vi "SimpleTokenizer.vi"() -> ()   [LabVIEW 2012]
uses:
  <vilib>/regexp/Match Regular Expression.xnode
panel:
  in  "Input String":string
  out "Next String Start":dbl
  out "Tokenized Array":string[](array[string])
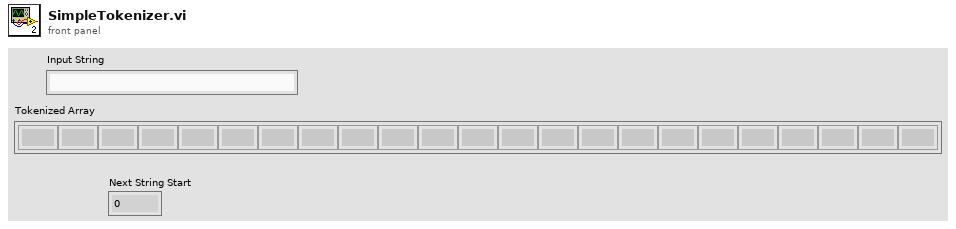
[diagram p1: front panel]
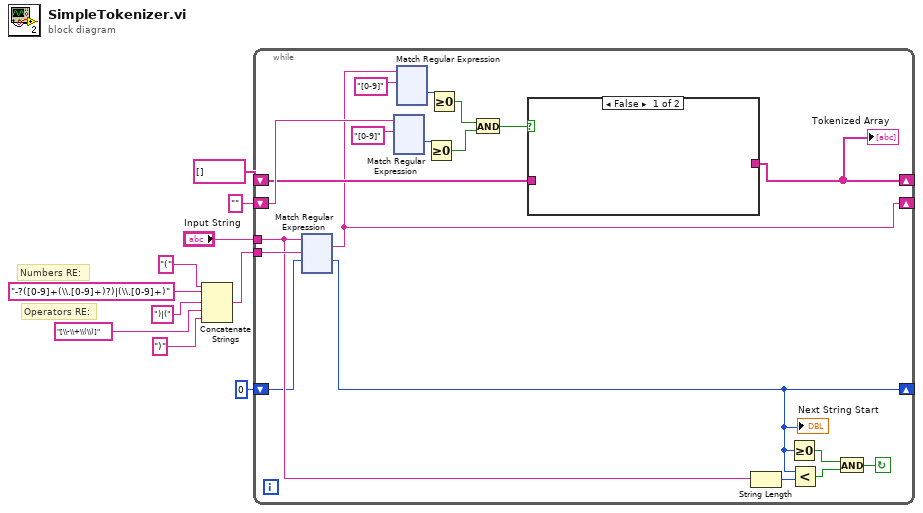
[diagram p0: block diagram]
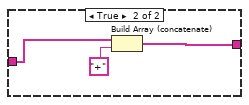
[diagram p2: hidden frame]
diagram:
  # "Operators RE:"
  # "Numbers RE:"
  n1 = Concatenate Strings("(", "-?([0-9]+(\\.[0-9]+)?)|(\\.[0-9]+)", ")|(", "[\\-\\+\\(\\)]", ")") -> (w4:string)
  n2 = while {
    shift-right: [w12] -> _
    shift-left: string[] [] -> [w13]
    shift-right: [w22] -> _
    shift-left: 0 ("offset (0)") -> [w27]
    tunnel: w4 -> [w29]
    shift-right: [w11] -> _
    shift-left: "" ("whole match") -> [w16]
    tunnel: "Input String" -> [w28]
    stop <- w26 continue-if-true
    n3 = xnode "Match Regular Expression"("input string"=w28, "regular expression"=w29, "offset (0)"=w27) -> ("whole match"=w11:string, "offset past match"=w22:i32)  [unwired: 3 in, 3 out]
    "Next String Start" <- w22
    n4 = xnode "Match Regular Expression"("input string"=w16, "regular expression"="[0-9]") -> ("offset past match"=w17:i32)  [unwired: 4 in, 4 out]
    n5 = xnode "Match Regular Expression"("input string"=w11, "regular expression"="[0-9]") -> ("offset past match"=w20:i32)  [unwired: 4 in, 4 out]
    n6 = Greater Or Equal To 0?(x=w17) -> (x >= 0?=w15:bool)
    n7 = Greater Or Equal To 0?(x=w20) -> (x >= 0?=w19:bool)
    n8 = And(x=w19, y=w15) -> (x .and. y?=w14:bool)
    n9 = case shown="False" w14 {
      tunnel: [_ w253] -> w12
      tunnel: w13 -> [_ w252]
      frame False {
      }
      frame True {
        n10 = Build Array (concatenate)(w252, "+") -> (w253:string[])
      }
    }
    "Tokenized Array" <- w12
    n11 = String Length(string=w28) -> (length=w23:i32)
    n12 = Greater Or Equal To 0?(x=w22) -> (x >= 0?=w25:bool)
    n13 = Less?(x=w22, y=w23) -> (x < y?=w24:bool)
    n14 = And(x=w25, y=w24) -> (x .and. y?=w26:bool)
  }
